vi "open.vi"(8 "error in (no error)":errorcluster, 10 "serial":string="alpaoLSDM88-25-001", 11 "SIMU_MIRROR in":refnum<class "SIMU_MIRROR.lvclass">) -> (0 "error out":errorcluster, 3 "SIMU_MIRROR out":refnum<class "SIMU_MIRROR.lvclass">)   [LabVIEW 2020, in "SIMU_MIRROR.lvclass"]
uses:
  SIMU_MIRROR.lvclass
  mirror.lvclass
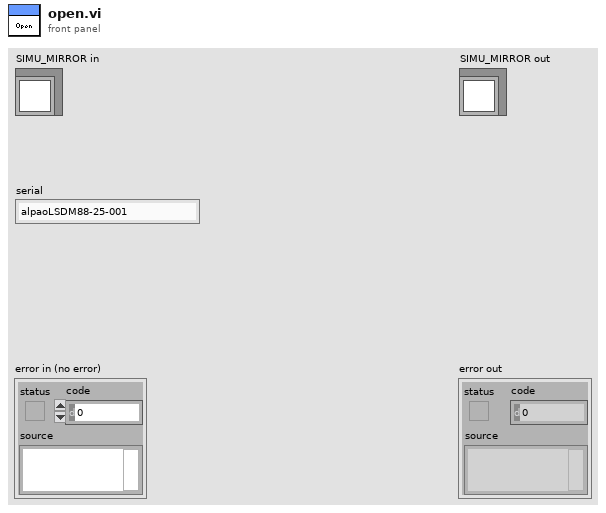
[diagram p1: front panel]
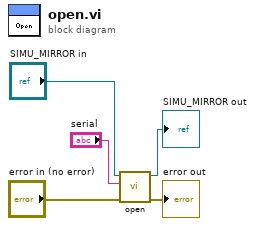
[diagram p0: block diagram]
diagram:
  n1 = call-parent "open.vi"("error in (no error)"="error in (no error)", "serial"="serial", "mirror in"="SIMU_MIRROR in") -> ("error out"=→"error out":errorcluster, "mirror out"=→"SIMU_MIRROR out":refnum<class "SIMU_MIRROR.lvclass">)  [unwired: 7 in]
